vi "Resolve Targets.vi"(10 "Target Group Maps":T1, 11 "Target ID":u32) -> (3 "Targets":u32[](array[numeric]))   [LabVIEW 2020, in "Vecto.lvlib" / "TCPMessaging.lvclass"]
uses:
  TCPMessaging.lvclass
  TCPMessaging.lvclass/TCPMessaging.ctl
  Target Group Maps.ctl
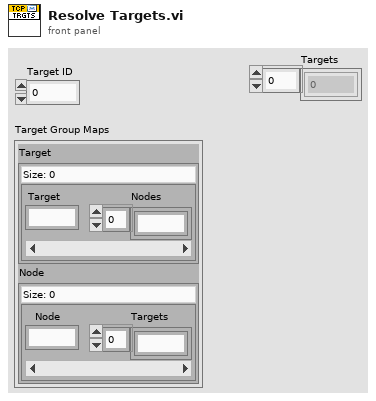
[diagram p1: front panel]
types:
  T1 = typedef "Vecto.lvlib/TCPMessaging.lvclass/Target Group Maps.ctl" = cluster{"Target":map{u32, u32[]}, "Node":map{u32, u32[]}}
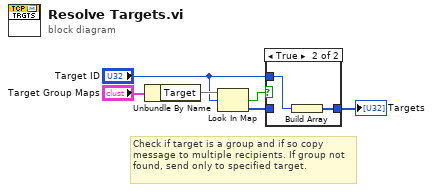
[diagram p0: block diagram]
diagram:
  # "Check if target is a group and if so copy message to multiple recipients. If group not found, send only to specified target."
  n1 = Unbundle By Name("Target Group Maps") -> ("Target"=w5:map{u32, u32[]})
  n2 = Look In Map(map=w5, key="Target ID") -> (key not found?=w4:bool, value=w3:u32[])  [unwired: 1 in]
  n3 = case shown="True" w4 {
    tunnel: w3 -> [w7 _]
    tunnel: [w7 w9] -> w2
    tunnel: "Target ID" -> [_ w8]
    frame False {
    }
    frame True {
      n4 = Build Array(w8) -> (w9:u32[])
    }
  }
  "Targets" <- w2
